vi "Execute.vi"(8 "error in (no error)":errorcluster, 11 "Node in":refnum<class "bt_Not.lvclass">) -> (0 "error out":errorcluster, 1 "Status":T1, 3 "Node out":refnum<class "bt_Not.lvclass">)   [LabVIEW 2021, in "BT.lvlib" / "bt_Not.lvclass"]
uses:
  bt_Not.lvclass
  bt_Not.lvclass/bt_Not.ctl
  abs_Node/Status.ctl
  abs_Node/bt_Node.lvclass
  Support/Decorator/bt_Decorator.lvclass
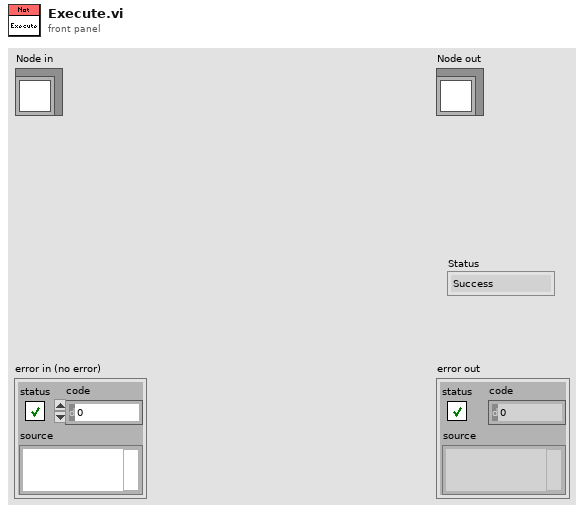
[diagram p1: front panel]
types:
  T1 = typedef "BT.lvlib/bt_Node.lvclass/Status.ctl" = enum16{"Success", "Failure", "Running"}
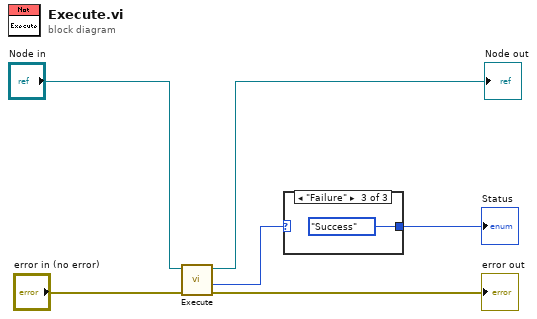
[diagram p0: block diagram]
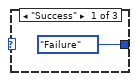
[diagram p2: hidden frame]
diagram:
  n1 = call-parent "Execute.vi"("error in (no error)"="error in (no error)", "Node in"="Node in") -> ("error out"=→"error out":errorcluster, "Status"=w1:T1, "Node out"=→"Node out":refnum<class "bt_Not.lvclass">)  [unwired: 7 in]
  n2 = case shown="\"Failure\"" w1 {
    selector: w1 -> [_ w8 _]
    tunnel: [Status."Failure" ("Status") w8 Status."Success" ("Status")] -> w2
    frame "Success" {
    }
    frame "Running" {
    }
    frame "Failure" {
    }
  }
  "Status" <- w2
